vi "Offset - minmax.vi"(1 "Offset":bool=TRUE, 2 "Pulse signal in":dbl[](array[numeric])) -> (6 "Pulse signal out":dbl[](array[numeric]))   [LabVIEW 2012]
panel:
  out "Pulse signal in graph out":dbl[](graph)
  out "Pulse signal in graph":dbl[](graph)
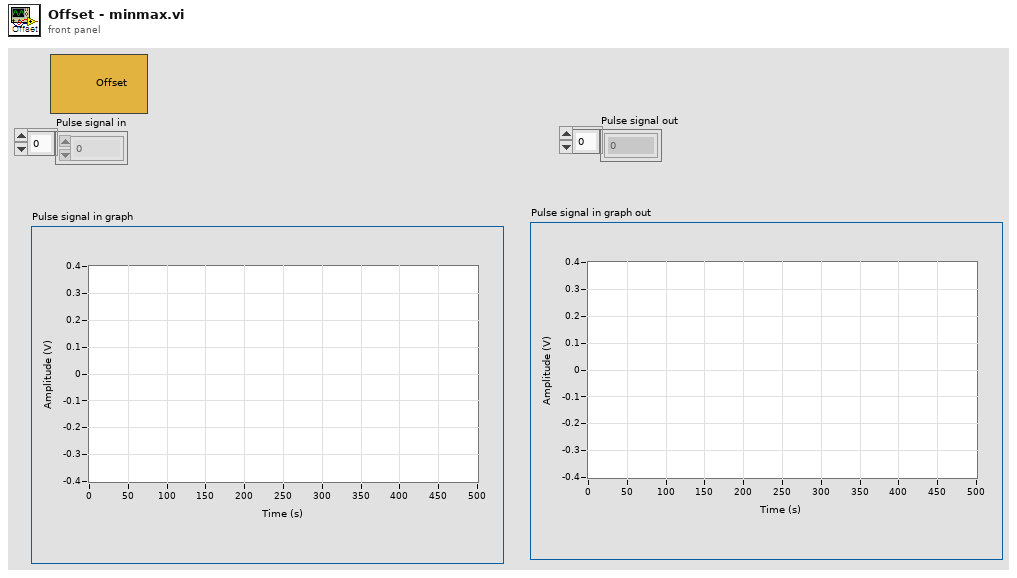
[diagram p1: front panel]
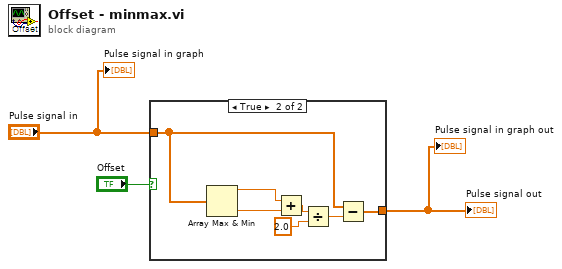
[diagram p0: block diagram]
diagram:
  n1 = case shown="True" "Offset" {
    tunnel: "Pulse signal in" -> [w4 w7]
    tunnel: [w4 w10] -> w2
    frame False {
    }
    frame True {
      n2 = Array Max & Min(array=w7) -> (max value=w6:dbl, min value=w5:dbl)  [unwired: 2 out]
      n3 = Add(x=w6, y=w5) -> (x+y=w11:dbl)
      n4 = Divide(x=w11, y=2.0) -> (x/y=w8:dbl)
      n5 = Subtract(x=w7, y=w8) -> (x-y=w10:dbl[])
    }
  }
  "Pulse signal out" <- w2
  "Pulse signal in graph out" <- w2
  "Pulse signal in graph" <- "Pulse signal in"
